vi "Temporizador.vi"(8 "error in":errorcluster, 10 "Reset buton":bool, 11 "Set Time":i16) -> (0 "error out":errorcluster, 2 "Next":bool, 3 "Sec":i16)   [LabVIEW 2023]
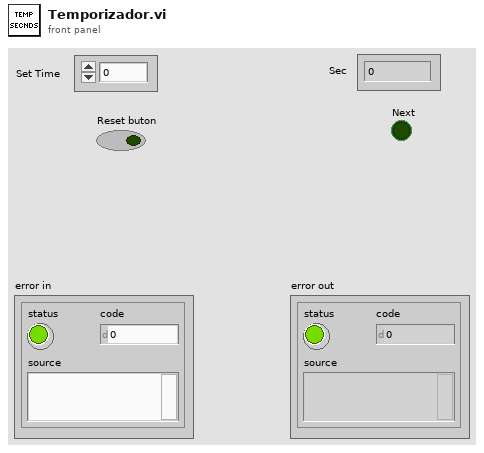
[diagram p1: front panel]
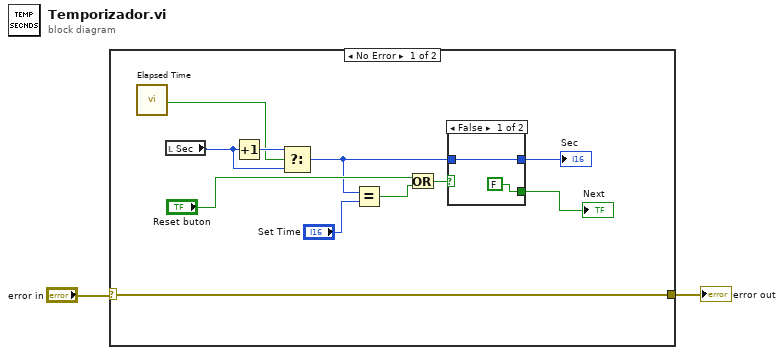
[diagram p0: block diagram]
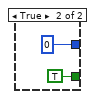
[diagram p2: hidden frame]
diagram:
  n1 = case shown="No Error" "error in" {
    selector: "error in" -> [w3 w18]
    tunnel: [w3 w18] -> w1
    frame No Error {
      n2 = call "Elapsed Time"() -> ("Time has Elapsed"=w7:bool)  [unwired: 12 in, 7 out]
      n3 = local read "Sec"() -> (w5:i16)
      n4 = Increment(x=w5) -> (x+1=w13:i16)
      n5 = Select(t=w13, s=w7, f=w5) -> (s? t:f=w4:i16)
      n6 = Equal?(x=w4, y="Set Time") -> (x = y?=w10:bool)
      n7 = Or(x="Reset buton", y=w10) -> (x .or. y?=w11:bool)
      n8 = case shown="False" w11 {
        tunnel: [w15 i16 0 ("Sec")] -> w6
        tunnel: w4 -> [w15 _]
        tunnel: [FALSE TRUE] -> w8
        frame False {
        }
        frame True {
        }
      }
      "Sec" <- w6
      "Next" <- w8
    }
    frame Error {
    }
  }
  "error out" <- w1
